vi "GenerateXYArmPathPolygon.vi"(1 "PointSpacing (in)":dbl, 2 "EndPoint":T1, 3 "StartPoint":T1) -> (0 "XYPathPoints":T1[](array[typedef]))   [LabVIEW 2018]
uses:
  TypeDefs/ArmAbsolutePosition.ctl
  ArgosLib/ArgosLib.lvlib
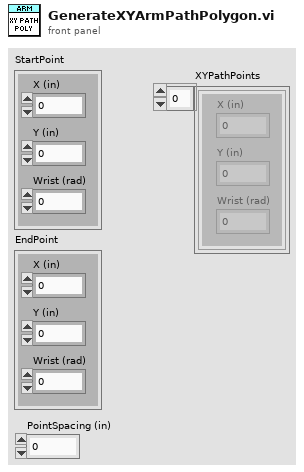
[diagram p1: front panel]
types:
  T1 = typedef "ArmAbsolutePosition.ctl" = cluster{"X (in)":dbl, "Y (in)":dbl, "Wrist (rad)":dbl}
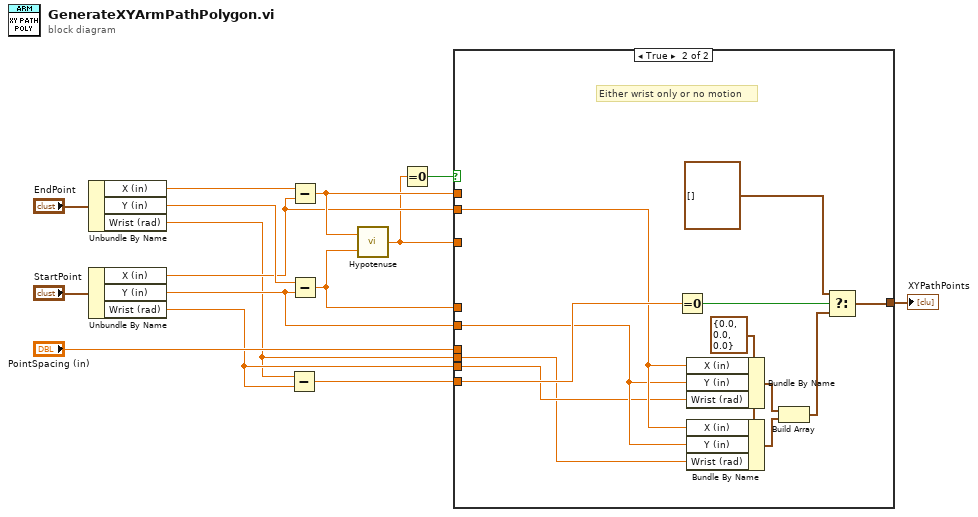
[diagram p0: block diagram]
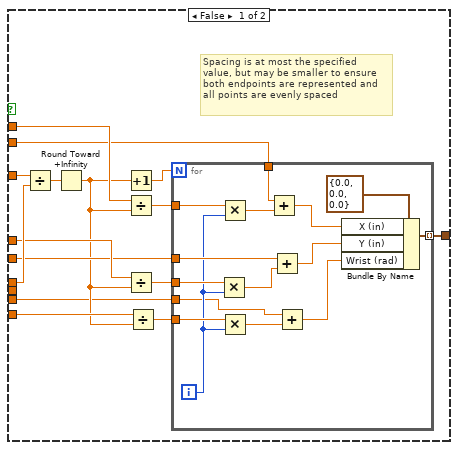
[diagram p2: hidden frame]
diagram:
  n1 = Unbundle By Name("EndPoint") -> ("X (in)"=w10:dbl, "Y (in)"=w9:dbl, "Wrist (rad)"=w1:dbl)
  n2 = Unbundle By Name("StartPoint") -> ("X (in)"=w8:dbl, "Y (in)"=w7:dbl, "Wrist (rad)"=w2:dbl)
  n3 = Subtract(x=w1, y=w2) -> (x-y=w3:dbl)
  n4 = Subtract(x=w10, y=w8) -> (x-y=w14:dbl)
  n5 = Subtract(x=w9, y=w7) -> (x-y=w13:dbl)
  n6 = call "Hypotenuse.vi"("Y"=w13, "X"=w14) -> ("Hypotenuse"=w5:dbl)
  n7 = Equal To 0?(x=w5) -> (x = 0?=w4:bool)
  n8 = case shown="True" w4 {
    tunnel: "PointSpacing (in)" -> [w30 _]
    tunnel: w14 -> [w26 _]
    tunnel: w13 -> [w25 _]
    tunnel: w8 -> [w24 w49]
    tunnel: w7 -> [w23 w48]
    tunnel: [w22 w50] -> w6
    tunnel: w5 -> [w20 _]
    tunnel: w3 -> [w19 w57]
    tunnel: w2 -> [w16 w47]
    tunnel: w1 -> [_ w46]
    frame False {
      # "Spacing is at most the specified\nvalue, but may be smaller to ensure\nboth endpoints are represented and\nall points are evenly spaced"
      n9 = Divide(x=w20, y=w30) -> (x/y=w29:dbl)
      n10 = Round Toward +Infinity(x=w29) -> (ceil(x): smallest int >= x=w18:dbl)
      n11 = Increment(x=w18) -> (x+1=w21:dbl)
      n12 = Divide(x=w26, y=w18) -> (x/y=w27:dbl)
      n13 = Divide(x=w25, y=w18) -> (x/y=w28:dbl)
      n14 = Divide(x=w19, y=w18) -> (x/y=w17:dbl)
      n15 = for {
        N: w21 -> [_]
        tunnel: w24 -> [w45]
        tunnel: w23 -> [w44]
        tunnel: w28 -> [w41]
        tunnel: w27 -> [w40]
        tunnel: [w36] -> w22 mode=indexing
        tunnel: w17 -> [w35]
        tunnel: w16 -> [w32]
        i -> [w34]
        n16 = Multiply(x=w41, y=w34) -> (x*y=w43:dbl)
        n17 = Multiply(x=w40, y=w34) -> (x*y=w42:dbl)
        n18 = Multiply(x=w35, y=w34) -> (x*y=w33:dbl)
        n19 = Add(x=w45, y=w42) -> (x+y=w38:dbl)
        n20 = Add(x=w44, y=w43) -> (x+y=w37:dbl)
        n21 = Add(x=w32, y=w33) -> (x+y=w31:dbl)
        n22 = Bundle By Name(cluster=T1 {"X (in)"=0.0, "Y (in)"=0.0, "Wrist (rad)"=0.0} ("2DPoint"), "X (in)"=w38, "Y (in)"=w37, "Wrist (rad)"=w31) -> (w36:T1)
      }
    }
    frame True {
      w54 = T1 {"X (in)"=0.0, "Y (in)"=0.0, "Wrist (rad)"=0.0} ("2DPoint")
      # "Either wrist only or no motion"
      n23 = Equal To 0?(x=w57) -> (x = 0?=w55:bool)
      n24 = Bundle By Name(cluster=w54, "X (in)"=w49, "Y (in)"=w48, "Wrist (rad)"=w47) -> (w53:T1)
      n25 = Bundle By Name(cluster=w54, "X (in)"=w49, "Y (in)"=w48, "Wrist (rad)"=w46) -> (w52:T1)
      n26 = Build Array(w53, w52) -> (w51:T1[])
      n27 = Select(t=T1[] [], s=w55, f=w51) -> (s? t:f=w50:T1[])
    }
  }
  "XYPathPoints" <- w6
